vi "GetVersion.vi"(8 "Error In":errorcluster) -> (0 "error out":errorcluster, 1 "Version Numbers":T1, 2 "Version String":string)   [LabVIEW 2020]
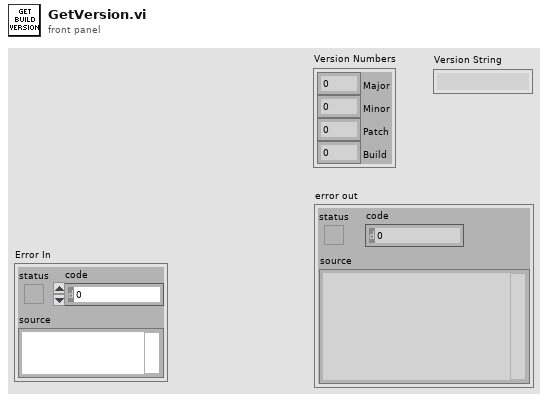
[diagram p1: front panel]
types:
  T1 = cluster{"Major":i32, "Minor":i32, "Patch":i32, "Build":i32}
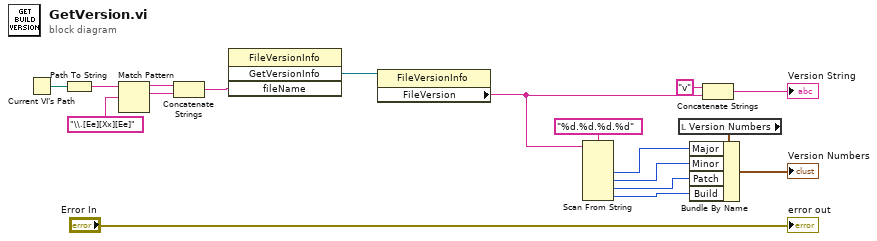
[diagram p0: block diagram]
diagram:
  n1 = Current VI's Path() -> (path=w9:path)
  n2 = Path To String(path=w9) -> (string=w4:string)
  n3 = Match Pattern(string=w4, regular expression="\\.[Ee][Xx][Ee]") -> (before substring=w6:string, match substring=w7:string)  [unwired: 1 in, 2 out]
  n4 = Concatenate Strings(w6, w7) -> (w5:string)
  n5 = invoke class="FileVersionInfo" method="GetVersionInfo"("fileName"=w5) -> ("GetVersionInfo"=w16:refnum<k24>)  [unwired: 3 in, 3 out]
  n6 = property class="FileVersionInfo"(reference=w16) -> ("FileVersion"=w2:string)  [unwired: 1 in, 2 out]
  n7 = Scan From String(format string="%d.%d.%d.%d", input string=w2) -> (output 1=w10:i32, output 2=w11:i32, output 3=w12:i32, output 4=w13:i32)  [unwired: 6 in, 3 out]
  n8 = local read "Version Numbers"() -> (w14:T1)
  n9 = Bundle By Name(cluster=w14, "Major"=w10, "Minor"=w11, "Patch"=w12, "Build"=w13) -> (→"Version Numbers":T1)
  n10 = Concatenate Strings("v" ("string"), w2) -> (→"Version String":string)
  "error out" <- "Error In"
